vi "UHR-Fleezers Control (host) - 12.5.vi"() -> ()   [LabVIEW 2012] (continued)
        n1392 = Multiply(x=w2006, y=3.2767) -> (x*y=w2005:dbl)
        n1393 = local read "Green Intensity % (FB OFF)"() -> (w2009:dbl)
        n1394 = Multiply(x=w2009, y=655.35) -> (x*y=w2010:dbl)
        n1395 = To Unsigned Word Integer(number=w2010) -> (unsigned 16bit integer=w2008:u16)
        n1396 = local read "Green int current ON count adj"() -> (w2012:u32)
        n1397 = local read "Laser interlacing mode"() -> (w2002:enum32{"Laser ON", "Laser OFF", "Interlace"})
        n1398 = local read "Green FB Gains"() -> (w1999:T9)
        n1399 = local read "Green Laser ON"() -> (w2003:bool)
        n1400 = local read "Green FB On/Off"() -> (w2013:bool)
        n1401 = Equal?(x=w2002, y=enum32{"Laser ON", "Laser OFF", "Interlace"}."Interlace") -> (x = y?=w2000:bool)
        n1402 = Unbundle By Name(w1999) -> ("proportional gain (Kc)"=w1998:i16, "integral gain (Kc*Ts/Ti)"=w1997:i16, "derivative gain (Kc*Td/Ts)"=w1996:i16)
        n1403 = Compound Arithmetic op=AND(w2000, w2013, w2003) -> (w2004:bool)
        n1404 = xnode "Read/Write Control"("FPGA VI Reference In"=w2016, "error in"=w2015, "Green FB Setpoint"=w2005, "Green FB On/Off"=w2004, "Current Out"=w2008, "Green int current ON count adj"=w2012, "P3"=w1998, "I3"=w1997, "D3"=w1996) -> ("error out"=w2014:errorcluster)  [unwired: 1 out]
      }
      event "Blue FB Setpoint (mV)", "Blue FB Gains", "Blue FB On/Off", "Blue Intensity % (FB OFF)", "Blue int AO ON count adjust": Value Change {
        # "16 bit analog out"
        n1405 = event-data() -> ()  [unwired: 7 out]
        n1406 = Multiply(x="Blue FB Setpoint (mV)", y=3.2767) -> (x*y=w2030:dbl)
        n1407 = Multiply(x="Blue Intensity % (FB OFF)", y=655.35) -> (x*y=w2033:dbl)
        n1408 = To Unsigned Word Integer(number=w2033) -> (unsigned 16bit integer=w2032:u16)
        n1409 = local read "Laser interlacing mode"() -> (w2028:enum32{"Laser ON", "Laser OFF", "Interlace"})
        n1410 = Unbundle By Name("Blue FB Gains") -> ("proportional gain (Kc)"=w2025:i16, "integral gain (Kc*Ts/Ti)"=w2024:i16, "derivative gain (Kc*Td/Ts)"=w2023:i16)
        n1411 = local read "Blue Laser ON"() -> (w2017:bool)
        n1412 = Equal?(x=w2028, y=enum32{"Laser ON", "Laser OFF", "Interlace"}."Interlace") -> (x = y?=w2026:bool)
        n1413 = Compound Arithmetic op=AND(w2026, "Blue FB On/Off", w2017) -> (w2029:bool)
        n1414 = xnode "Read/Write Control"("FPGA VI Reference In"=w2037, "error in"=w2036, "Blue FB Setpoint"=w2030, "Blue FB On/Off"=w2029, "BI Current Out"=w2032, "Blue current ON count adj (AO)"="Blue int AO ON count adjust", "P5"=w2025, "I5"=w2024, "D5"=w2023) -> ("error out"=w2035:errorcluster)  [unwired: 1 out]
      }
      event "Red FB Setpoint (mV)", "Red FB Gains", "Red FB On/Off", "Red Intensity % (FB OFF)", "Red int current ON count adj": Value Change {
        n1415 = event-data() -> ()  [unwired: 7 out]
        n1416 = local read "Red FB Setpoint (mV)"() -> (w2049:dbl)
        n1417 = Multiply(x=w2049, y=3.2767) -> (x*y=w2048:dbl)
        n1418 = local read "Red Intensity % (FB OFF)"() -> (w2038:dbl)
        n1419 = Multiply(x=w2038, y=655.35) -> (x*y=w2052:dbl)
        n1420 = To Unsigned Word Integer(number=w2052) -> (unsigned 16bit integer=w2051:u16)
        n1421 = local read "Red int current ON count adj"() -> (w2054:u16)
        n1422 = local read "Laser interlacing mode"() -> (w2045:enum32{"Laser ON", "Laser OFF", "Interlace"})
        n1423 = local read "Red FB Gains"() -> (w2042:T9)
        n1424 = local read "Red Laser ON"() -> (w2046:bool)
        n1425 = local read "Red FB On/Off"() -> (w2055:bool)
        n1426 = Equal?(x=w2045, y=enum32{"Laser ON", "Laser OFF", "Interlace"}."Interlace") -> (x = y?=w2043:bool)
        n1427 = Unbundle By Name(w2042) -> ("proportional gain (Kc)"=w2041:i16, "integral gain (Kc*Ts/Ti)"=w2040:i16, "derivative gain (Kc*Td/Ts)"=w2039:i16)
        n1428 = Compound Arithmetic op=AND(w2043, w2055, w2046) -> (w2047:bool)
        n1429 = xnode "Read/Write Control"("FPGA VI Reference In"=w2058, "error in"=w2057, "Red FB Setpoint"=w2048, "Red FB On/Off"=w2047, "RI Current Out"=w2051, "Red int current ON count adj"=w2054, "P4"=w2041, "I4"=w2040, "D4"=w2039) -> ("error out"=w2056:errorcluster)  [unwired: 1 out]
      }
      event "+ phase (APD 1 Gate)", "- phase (APD 1 Gate)", "+ phase (APD 2 Gate)", "- phase (APD 2 Gate)", "+ phase (APD 3 Gate)", "- phase (APD 3 Gate)", "+ phase (APD Acq)", "- phase (APD Acq)": Value Change {
        n1430 = event-data() -> ()  [unwired: 7 out]
        n1431 = local read "Phase Adj. (APD 1 Gate)"() -> (w2078:i16)
        n1432 = Or(x="- phase (APD 1 Gate)", y="+ phase (APD 1 Gate)") -> (x .or. y?=w2080:bool)
        n1433 = Negate(x=w2078) -> (-x=w2085:i16)
        n1434 = Select(t=w2085, s="+ phase (APD 1 Gate)", f=w2078) -> (s? t:f=w2084:i16)
        n1435 = local read "Phase Adj. (APD 2 Gate)"() -> (w2075:i16)
        n1436 = Or(x="- phase (APD 2 Gate)", y="+ phase (APD 2 Gate)") -> (x .or. y?=w2073:bool)
        n1437 = Negate(x=w2075) -> (-x=w2077:i16)
        n1438 = Select(t=w2077, s="+ phase (APD 2 Gate)", f=w2075) -> (s? t:f=w2074:i16)
        n1439 = Negate(x="Phase Adj. (APD 3 Gate)") -> (-x=w2072:i16)
        n1440 = Or(x="- phase (APD 3 Gate)", y="+ phase (APD 3 Gate)") -> (x .or. y?=w2068:bool)
        n1441 = Select(t=w2072, s="+ phase (APD 3 Gate)", f="Phase Adj. (APD 3 Gate)") -> (s? t:f=w2069:i16)
        n1442 = local read "Phase Adj. (APD Acq)"() -> (w2066:i16)
        n1443 = Or(x="- phase (APD Acq)", y="+ phase (APD Acq)") -> (x .or. y?=w2064:bool)
        n1444 = Negate(x=w2066) -> (-x=w2067:i16)
        n1445 = Select(t=w2067, s="+ phase (APD Acq)", f=w2066) -> (s? t:f=w2065:i16)
        n1446 = xnode "Read/Write Control"("FPGA VI Reference In"=w2087, "error in"=w2086, "Phase count adjustment (APD 1 Gate)"=w2084, "Phase count adjustment (APD 2 Gate)"=w2074, "Phase count adjustment (APD 3 Gate)"=w2069, "Phase Count Adjustment (APD Acq)"=w2065) -> ("FPGA VI Reference Out"=w2082:T20, "error out"=w2083:errorcluster)
        n1447 = xnode "Read/Write Control"("FPGA VI Reference In"=w2082, "error in"=w2083, "+ phase (APD 1 Gate)"=w2080, "+ phase (APD 2 Gate)"=w2073, "+ phase (APD 3 Gate)"=w2068, "+ phase (APD Acq)"=w2064) -> ("error out"=w2081:errorcluster)  [unwired: 1 out]
      }
      event "Invert APD Gate", "APD Gate ON Count", "APD Gate OFF Count", "APD Gate", "APD Integration Time (s)", "APD AO Scale Factor", "Duty Frequency (ON 1/N cycles)", "Interlace ON count", "Interlace OFF count": Value Change {
        n1448 = event-data() -> ()  [unwired: 7 out]
        n1449 = Add(x="Interlace ON count", y="Interlace OFF count") -> (x+y=w2093:u16)
        n1450 = Add(x="APD Gate ON Count", y="APD Gate OFF Count") -> (x+y=w2104:u16)
        n1451 = Multiply(x="Duty Frequency (ON 1/N cycles)", y=w2093) -> (x*y=w2089:u16)
        "Green AI Count" <- w2089
        "Red AI Count" <- w2089
        "Blue AI Count" <- w2089
        n1452 = Subtract(x=w2089, y="Interlace ON count") -> (x-y=w2092:u16)
        n1453 = Multiply(x=w2104, y="Duty Frequency (ON 1/N cycles)") -> (x*y=w2103:u16)
        n1454 = Subtract(x=w2103, y="APD Gate ON Count") -> (x-y=w2102:u16)
        n1455 = local read "DMA Update Period (s)"() -> (w2105:dbl)
        n1456 = Multiply(x="APD Integration Time (s)", y=40000000.0) -> (x*y=w2109:dbl)
        n1457 = Reciprocal(x="APD Integration Time (s)") -> (1/x=→"APD Acq Rate (Hz)":dbl)
        n1458 = To Unsigned Long Integer(number=w2109) -> (unsigned 32bit integer=w2095:u32)
        "APD Int. Count" <- w2095
        n1459 = local read "Number of APDs"() -> (w2088:u8)
        n1460 = Divide(x=w2105, y="APD Integration Time (s)") -> (x/y=w2107:dbl)
        n1461 = Multiply(x=w2088, y=w2107) -> (x*y=w2106:dbl)
        n1462 = local write "APD Samples/FIFO Acq."(w2107) -> ()
        n1463 = local write "APD Elements/DMA read"(w2106) -> ()
        n1464 = xnode "Read/Write Control"("FPGA VI Reference In"=w2113, "error in"=w2112, "Invert APD Gate"="Invert APD Gate", "APD Gate ON Count"="APD Gate ON Count", "APD Gate OFF Count"=w2102, "APD Acq Rate Count"=w2095, "APD Gate Operating Mode"="APD Gate", "APD AO scale factor"="APD AO Scale Factor", "Green interlace ON count"="Interlace ON count", "Green interlace OFF count"=w2092, "Green interlace ON count 2"="Interlace ON count", "Green interlace OFF count 2"=w2092, "Green FB Count"=w2089, "Red interlace ON count"="Interlace ON count", "Red interlace OFF count"="Interlace OFF count", "Red FB Count"=w2089, "Red interlace ON count 2"="Interlace ON count", "Red interlace OFF count 2"="Interlace OFF count", "Blue ON count (AO)"="Interlace ON count", "Blue OFF count (AO)"="Interlace OFF count", "Blue interlace OFF count (D)"="Interlace OFF count", "Blue interlace ON count (D)"="Interlace ON count", "Blue Int Count"=w2089) -> ("error out"=w2111:errorcluster)  [unwired: 1 out]
      }
      event "Neg. TTrig FPGA": Value Change {
        n1465 = event-data() -> ()  [unwired: 7 out]
        n1466 = xnode "Read/Write Control"("FPGA VI Reference In"=w2116, "error in"=w2115, "TTrig Negate Pos"="Neg. TTrig FPGA") -> ()  [unwired: 2 out]
      }
      event "Test ttrig": Value Change {
        n1467 = event-data() -> ()  [unwired: 7 out]
        n1468 = xnode "Read/Write Control"("FPGA VI Reference In"=w2120, "error in"=w2119, "TTrig?"=TRUE) -> ("error out"=w2118:errorcluster)  [unwired: 1 out]
      }
      event "Number of F/B Scans (AOD)", "Scan Speed (nm/s)", "Scan BD", "Initial delta (MHz)", "Step Size (nm)", "Scan Range (nm)": Value Change {
        w2183 = 123.0  # AOM cal (nm/MHz)
        n1469 = event-data() -> ()  [unwired: 7 out]
        n1470 = local read "BD 1 Frequency 1 (MHz)"() -> (w2166:dbl)
        n1471 = local read "AOM X Cal (nm/MHz)"() -> (w2158:dbl)
        n1472 = local read "X RF Frequency Limits (MHz)"() -> (w2170:T16)
        n1473 = local read "Y RF Frequency Limits (MHz)"() -> (w2167:T16)
        n1474 = local read "BD 2 Frequency 1 (MHz)"() -> (w2172:dbl)
        n1475 = Negate(x="Scan Range (nm)") -> (-x=w2136:dbl)
        n1476 = Divide(x=w2136, y=w2158) -> (x/y=w2140:dbl)
        n1477 = Select(t=w2170, s="Scan BD", f=w2167) -> (s? t:f=w2169:T16)
        n1478 = Select(t=w2166, s="Scan BD", f=w2172) -> (s? t:f=w2171:dbl)
        n1479 = Unbundle By Name(w2169) -> ("Maximum"=w2178:dbl, "Minimum"=w2177:dbl)
        n1480 = Add(x=w2140, y=w2171) -> (x+y=w2175:dbl)
        n1481 = Divide(x=w2136, y="Step Size (nm)") -> (x/y=w2155:dbl)
        n1482 = Divide(x="Step Size (nm)", y=w2158) -> (x/y=w2164:dbl)
        n1483 = Absolute Value(x=w2155) -> (abs(x)=w2139:dbl)
        n1484 = Sign(1:w2136) -> (0:w2137:dbl)
        n1485 = In Range and Coerce(upper limit=w2178, x=w2175, lower limit=w2177) -> (coerced(x)=w2174:dbl, In Range?=w2176:bool)
        n1486 = To Unsigned Quad Integer(1:w2139) -> (0:w2154:u64)
        "Scan steps (AOD)" <- w2154
        n1487 = call "IR AOM freq to word.vi"("Frequency In (MHz)"=w2164) -> ("Frequency Word Out (double)"=w2161:dbl)
        n1488 = Multiply(x=w2137, y=w2161) -> (x*y=w2138:dbl)
        n1489 = Subtract(x=w2175, y=w2174) -> (x-y=w2173:dbl)
        n1490 = To Quad Integer(1:w2138) -> (0:w2160:i64)
        "Incr. int (AOD)" <- w2160
        n1491 = Subtract(x=w2140, y=w2173) -> (x-y=w2159:dbl)
        "Scan Range (MHz)" <- w2159
        n1492 = Select(t=w2140, s=w2176, f=w2159) -> (s? t:f=w2179:dbl)
        n1493 = Multiply(x=w2159, y=w2158) -> (x*y=w2157:dbl)
        n1494 = Decrement(x=w2154) -> (x-1=w2207:u64)
        n1495 = Negate(x=w2157) -> (-x=w2153:dbl)
        n1496 = local write "Scan Range (nm)"(w2153) -> ()
        n1497 = Divide(x=w2179, y=w2207) -> (x/y=w2163:dbl)
        "Scan Increment (MHz)" <- w2163
        n1498 = call "IR AOM freq to word.vi"("Frequency In (MHz)"=w2163) -> ("Frequency Word Out (double)"=w2162:dbl)
        n1499 = Divide(x="Step Size (nm)", y="Scan Speed (nm/s)") -> (x/y=w2150:dbl)
        n1500 = To Quad Integer(1:w2162) -> ()  [unwired: 1 out]
        n1501 = local read "Number Interlace Sets"() -> (w2134:u8)
        n1502 = local read "AI Count (ticks)"() -> (w2135:u16)
        n1503 = local read "Total Counts (ticks)"() -> (w2133:u16)
        n1504 = local read "# Samples/trap"() -> (w2165:u32)
        n1505 = Multiply(x=w2135, y=w2134) -> (x*y=w2132:u16)
        n1506 = Divide(x=w2133, y=w2132) -> (x/y=w2131:dbl)
        n1507 = Select(t=w2166, s="Scan BD", f=w2172) -> (s? t:f=w2204:dbl)
        "Initial freq. (MHz)" <- w2204
        n1508 = Add(x=w2179, y=w2204) -> (x+y=→"Final freq. (MHz)":dbl)
        n1509 = Divide(x=w2133, y=40000000.0) -> (x/y=w2149:dbl)
        n1510 = Divide(x=w2150, y=w2149) -> (x/y=w2148:dbl)
        n1511 = To Unsigned Quad Integer(1:w2148) -> (0:w2123:u64)
        n1512 = Quotient & Remainder(x=w2123, y=u64 2) -> (x-y*floor(x/y)=w2127:u64)  [unwired: 1 out]
        n1513 = Equal?(x=w2127, y=u64 0) -> (x = y?=w2125:bool)
        n1514 = Decrement(x=w2123) -> (x-1=w2124:u64)
        n1515 = Select(t=w2123, s=w2125, f=w2124) -> (s? t:f=w2122:u64)
        "Cycles/step (AOD)" <- w2122
        n1516 = xnode "Read/Write Control"("FPGA VI Reference In"=w2215, "error in"=w2214, "Scan steps"=w2154, "Number of scans"="Number of F/B Scans (AOD)", "Cycles per step"=w2122, "Scan freq.  increment"=w2160, "Scan BD"="Scan BD") -> ("error out"=w2213:errorcluster)  [unwired: 1 out]
        n1517 = Multiply(x=w2154, y=w2122) -> (x*y=w2208:u64)
        n1518 = Multiply(x=w2208, y=u64 2) -> (x*y=w2130:u64)
        n1519 = Multiply(x=w2131, y=w2130) -> (x*y=w2129:dbl)
        "Data points/scan (f/b)" <- w2129
        n1520 = Multiply(x=w2129, y="Number of F/B Scans (AOD)") -> (x*y=w2211:dbl)
        "Data points/scans" <- w2211
        n1521 = Divide(x=w2211, y=w2165) -> (x/y=→"N sets should be saved":dbl)
        n1522 = Multiply(x=w2208, y=w2149) -> (x*y=w2147:dbl)
        "Time/Scan (s) (AOD)" <- w2147
        n1523 = Select(t=w2179, s="Scan BD", f=0.0) -> (s? t:f=w2205:dbl)
        n1524 = Select(t=0.0, s="Scan BD", f=w2179) -> (s? t:f=w2201:dbl)
        n1525 = local read "BD 2 Frequency 2 (MHz)"() -> (w2197:dbl)
        n1526 = local read "BD 1 Frequency 2 (MHz)"() -> (w2200:dbl)
        n1527 = Add(x=w2201, y=w2172) -> (x+y=w2198:dbl)
        n1528 = Add(x=w2166, y=w2205) -> (x+y=w2199:dbl)
        n1529 = Multiply(x=w2147, y=2.0) -> (x*y=w2146:dbl)
        n1530 = Multiply(x=w2146, y="Number of F/B Scans (AOD)") -> (x*y=w2143:dbl)
        n1531 = Divide(x=w2143, y=60.0) -> (x/y=→"Time to Finish All (min)":dbl)
        n1532 = Add(x="Trap 2 Bead Size (nm)", y="Trap 1 Bead Size (nm)") -> (x+y=w2187:dbl)
        n1533 = Divide(x=w2187, y=2.0) -> (x/y=w2181:dbl)
        n1534 = local read "Initial delta (MHz)"() -> (w2184:dbl)
        n1535 = Subtract(x=w2198, y=w2197) -> (x-y=w2195:dbl)
        n1536 = Subtract(x=w2199, y=w2200) -> (x-y=w2196:dbl)
        n1537 = Square(x=w2195) -> (x^2=w2194:dbl)
        n1538 = Square(x=w2196) -> (x^2=w2193:dbl)
        n1539 = Add(x=w2193, y=w2194) -> (x+y=w2192:dbl)
        n1540 = Square Root(x=w2192) -> (sqrt(x)=w2191:dbl)
        "Final delta (MHz)" <- w2191
        n1541 = Multiply(x=w2183, y=w2191) -> (x*y=w2190:dbl)
        n1542 = Multiply(x=w2184, y=w2183) -> (x*y=w2182:dbl)
        n1543 = Subtract(x=w2182, y=w2181) -> (x-y=→"Initial sep (nm)":dbl)
        n1544 = Subtract(x=w2190, y=w2181) -> (x-y=→"Final sep (nm)":dbl)
      }
      event "Freq or Amp switch first", "Swap F1 and F2", "Freq switch delay", "Amp switch delay": Value Change {
        n1545 = event-data() -> ()  [unwired: 7 out]
        n1546 = local read "Amp switch delay"() -> (w2216:u16)
        n1547 = local read "Swap F1 and F2"() -> (w2217:bool)
        n1548 = xnode "Read/Write Control"("FPGA VI Reference In"=w2220, "error in"=w2219, "Swap F1 and F2"=w2217, "Amp switch delay"=w2216) -> ("error out"=w2218:errorcluster)  [unwired: 1 out]
      }
      event "Scan steps (MCL)", "Number of scans (MCL)", "Scan Range (V)\n(of steps)", "2D or 1D Scan", "N APD Samp/step", "Fast Scan Dir", "Continuous MCL Scanning", "Scan lines (y)": Value Change {
        w2222 = 32767.0 ("y")
        n1549 = event-data() -> ()  [unwired: 7 out]
        n1550 = Select(t="Scan lines (y)", s="2D or 1D Scan", f="Number of scans (MCL)") -> (s? t:f=w2227:u64)
        n1551 = Decrement(x="Scan steps (MCL)") -> (x-1=w2243:u64)
        n1552 = Divide(x="Scan Range (V)\n(of steps)", y=w2243) -> (x/y=w2242:dbl)
        "Desired Scan Incr (V)" <- w2242
        n1553 = local read "APD Integration Time (s)"() -> (w2235:dbl)
        n1554 = Multiply(x=w2242, y=w2222) -> (x*y=w2251:dbl)
        n1555 = Divide(x=w2251, y=10.0) -> (x/y=w2241:dbl)
        "Desired incr (int)" <- w2241
        n1556 = local read "Update Count (MCL)"() -> (w2247:u32)
        n1557 = Round Toward -Infinity(1:w2241) -> (0:w2250:dbl)
        n1558 = To Word Integer(number=w2250) -> (16bit integer=w2225:i16)
        "Actual Incr. int (MCL)" <- w2225
        n1559 = Multiply(x=w2235, y=40000000.0) -> (x*y=w2248:dbl)
        n1560 = Divide(x=w2248, y=w2247) -> (x/y=w2246:dbl)
        n1561 = Multiply(x=i16 10, y=w2225) -> (x*y=w2223:i16)
        n1562 = Multiply(x="N APD Samp/step", y=w2246) -> (x*y=w2245:dbl)
        "Cycles/step (MCL)" <- w2245
        n1563 = Divide(x=w2223, y=w2222) -> (x/y=→"Actual MCL Inc (V)":dbl)
        n1564 = Multiply(x="N APD Samp/step", y="Scan steps (MCL)") -> (x*y=w2237:dbl)
        n1565 = local read "APD Samples/FIFO Acq."() -> (w2234:dbl)
        n1566 = Multiply(x=w2237, y=u64 2) -> (x*y=w2236:dbl)
        "Data points/scan (f+b)" <- w2236
        n1567 = Multiply(x=w2236, y=w2227) -> (x*y=w2254:dbl)
        "Data points/scans (MCL)" <- w2254
        n1568 = Multiply(x=w2235, y=w2236) -> (x*y=w2228:dbl)
        "Time/f+b scan (s) (MCL)" <- w2228
        n1569 = Divide(x=w2254, y=w2234) -> (x/y=→"N sets should be saved (MCL)":dbl)
        n1570 = Multiply(x=w2228, y=w2227) -> (x*y=→"Total Time (s)":dbl)
        n1571 = Not(x="Fast Scan Dir") -> (.not. x?=w2232:bool)
        n1572 = xnode "Read/Write Control"("FPGA VI Reference In"=w2258, "error in"=w2257, "Scan steps (MCL)"="Scan steps (MCL)", "Number of scans (MCL)"=w2227, "Cycles per step (MCL)"=w2245, "Scan freq.  increment (MCL)"=w2225, "1D or 2D Scan?"="2D or 1D Scan", "MCL Scan Axis"=w2232, "Cont. Scan (MCL)"="Continuous MCL Scanning") -> ("error out"=w2256:errorcluster)  [unwired: 1 out]
      }
      event "Read Cal": Value Change {
        w2260 = 1000.0 ("y")
        n1573 = event-data() -> ()  [unwired: 7 out]
        n1574 = local read "Save file name"() -> (w2285:path)
        n1575 = local write "Read Cal"(FALSE ("Read Cal")) -> ()
        n1576 = Strip Path(path=w2285) -> (stripped path=w2284:path)  [unwired: 1 out]
        n1577 = Path To String(path=w2284) -> (string=w2283:string)
        n1578 = Concatenate Strings(w2283, "\\current.cal" ("string")) -> (w2281:string)
        n1579 = String To Path(string=w2281) -> (path=w2280:path)
        n1580 = Open/Create/Replace File(file path (use dialog)=w2280, operation (0:open)=T28."open", access (0:read/write)=enum16{"read/write", "read-only", "write-only"}."read-only") -> (refnum out=w2288:refnum<file>, error out=w2274:errorcluster)  [unwired: 1 in, 3 out]
        n1581 = Deny Access(4:w2274, 7:w2288) -> (0:w2273:errorcluster, 3:w2279:refnum<file>)  [unwired: 1 out]
        n1582 = Read from Binary File(5:0.0, 8:w2273, 9:T27."big-endian, network order" ("byte order (0:big-endian, network order)"), 10:-1 ("count (1)"), 11:w2279) -> (0:w2272:errorcluster, 2:w2270:dbl[], 3:w2275:refnum<file>)  [unwired: 2 out]
        n1583 = Array To Cluster(array=w2270) -> (cluster=w2269:T30)
        n1584 = Unbundle(w2269) -> ("[0]"=w2268:dbl, "[1]"=w2267:dbl, "[2]"=w2266:dbl, "[3]"=w2265:dbl, "[4]"=w2264:dbl, "[5]"=w2263:dbl)
        n1585 = Close File(refnum=w2275, error in=w2272) -> (error out=→"Read cal error":errorcluster)  [unwired: 1 out]
        n1586 = Multiply(x=w2263, y=w2260) -> (x*y=w2261:dbl)
        n1587 = local write "T2 kappa_x (pN/nm)"(w2265) -> ()
        n1588 = local write "T1 kappa_x (pN/nm)"(w2266) -> ()
        n1589 = local write "T1 alpha_x (nm/V)"(w2268) -> ()
        n1590 = local write "T2 alpha_x (nm/V)"(w2267) -> ()
        n1591 = Multiply(x=w2264, y=w2260) -> (x*y=w2262:dbl)
        n1592 = local write "T1 offset_x (mV)"(w2262) -> ()
        n1593 = local write "T2 offset_x (mV)"(w2261) -> ()
      }
      event "Abort MCL Scan": Value Change {
        n1594 = event-data() -> ()  [unwired: 7 out]
        n1595 = local write "MCL Scanning"(FALSE ("MCL Scanning")) -> ()
        n1596 = xnode "Read/Write Control"("FPGA VI Reference In"=w2293, "error in"=w2292, "Abort scan (MCL)"="Abort MCL Scan") -> ("error out"=w2291:errorcluster)  [unwired: 1 out]
      }
      event "Update Count (MCL)": Value Change {
        n1597 = event-data() -> ()  [unwired: 7 out]
        n1598 = xnode "Read/Write Control"("FPGA VI Reference In"=w2297, "error in"=w2296, "MCL count"="Update Count (MCL)") -> ("error out"=w2295:errorcluster)  [unwired: 1 out]
      }
      event "+ phase (MCL)", "- phase (MCL)": Value Change {
        n1599 = event-data() -> ()  [unwired: 7 out]
        n1600 = Or(x="- phase (MCL)", y="+ phase (MCL)") -> (x .or. y?=w2300:bool)
        n1601 = Negate(x="Phase adjust (MCL)") -> (-x=w2306:i16)
        n1602 = Select(t=w2306, s="+ phase (MCL)", f="Phase adjust (MCL)") -> (s? t:f=w2304:i16)
        n1603 = xnode "Read/Write Control"("FPGA VI Reference In"=w2308, "error in"=w2307, "Phase count adjustment (MCL)"=w2304) -> ("FPGA VI Reference Out"=w2301:T20, "error out"=w2302:errorcluster)
        n1604 = xnode "Read/Write Control"("FPGA VI Reference In"=w2301, "error in"=w2302, "+ phase (MCL)"=w2300) -> ("error out"=w2299:errorcluster)  [unwired: 1 out]
      }
      event "Abort AOD Scan": Value Change {
        n1605 = event-data() -> ()  [unwired: 7 out]
        n1606 = xnode "Read/Write Control"("FPGA VI Reference In"=w2312, "error in"=w2311, "Abort scan"="Abort AOD Scan") -> ("error out"=w2310:errorcluster)  [unwired: 1 out]
      }
      event "Continuous AOD Scanning": Value Change {
        n1607 = event-data() -> ()  [unwired: 7 out]
        n1608 = xnode "Read/Write Control"("FPGA VI Reference In"=w2316, "error in"=w2315, "Cont. Scan"="Continuous AOD Scanning") -> ("error out"=w2314:errorcluster)  [unwired: 1 out]
      }
      event "Index": Value Change {
        n1609 = event-data() -> ()  [unwired: 7 out]
        n1610 = call "Create new save file.vi"("Insert"="", "Ext"=".dat" ("string"), "Index In"="Index") -> ("Path Out"=→"Save file name":path, "Index Out"=w2317:dbl)
        "Save index" <- w2317
        n1611 = local write "Index"(w2317) -> ()
      }
      event "AO1", "AO2": Value Change {
        w2332 = 10.0 ("y")
        w2331 = 32767.0 ("y")
        n1612 = event-data() -> ()  [unwired: 7 out]
        n1613 = local read "AO2"() -> (w2330:dbl)
        n1614 = local read "AO1"() -> (w2327:dbl)
        n1615 = Multiply(x=w2327, y=w2331) -> (x*y=w2326:dbl)
        n1616 = Multiply(x=w2330, y=w2331) -> (x*y=w2329:dbl)
        n1617 = Divide(x=w2326, y=w2332) -> (x/y=w2325:dbl)
        n1618 = Divide(x=w2329, y=w2332) -> (x/y=w2328:dbl)
        n1619 = To Word Integer(number=w2325) -> (16bit integer=w2333:i16)
        n1620 = To Word Integer(number=w2328) -> (16bit integer=w2334:i16)
        n1621 = xnode "Read/Write Control"("FPGA VI Reference In"=w2324, "error in"=w2323, "AO1"=w2333, "AO2"=w2334) -> ("error out"=w2322:errorcluster)  [unwired: 1 out]
      }
      event "Inject Pump 1": Value Change {
        n1622 = event-data() -> ()  [unwired: 7 out]
        n1623 = local read "Use Harvard pumps\nfor beads (else Chemyx)"() -> (w2336:bool)
        n1624 = case shown="True" w2336 {
          tunnel: "Inject Pump 1" -> [w2340 w2378]
          tunnel: w2335 -> [_ w2379]
          frame False {
            n1625 = local read "Pump write delay (ms)"() -> (w2339:dbl)
            n1626 = local read "Chemyx Syringe Pump Serial Port"() -> (w2338:refnum<visa-resource-name>)
            n1627 = case shown="True" w2340 {
              tunnel: w2339 -> [w2346 w2360]
              tunnel: w2338 -> [w2343 w2359]
              frame False {
                n1628 = flat-sequence {
                  tunnel: w2343 -> [w2347]
                  tunnel: [w2347] -> w2344
                  tunnel: w2346 -> [_]
                  tunnel: [w2350] -> w2345
                  tunnel: w2344 -> [w2350]
                  tunnel: w2345 -> [w2351]
                  tunnel: [w2351] -> w2341
                  tunnel: [w2353] -> w2342
                  tunnel: w2341 -> [w2353]
                  tunnel: w2342 -> [w2355]
                  frame #0 {
                    n1629 = call "Write to pump.vi"("string"="enter pump1", "VISA resource name"=w2347) -> ()  [unwired: 1 out]
                  }
                  frame #1 {
                    n1630 = Wait (ms)(milliseconds to wait="Pump pause delay (ms)") -> ()  [unwired: 1 out]
                  }
                  frame #2 {
                    n1631 = call "Write to pump.vi"("string"="stop", "VISA resource name"=w2351) -> ()  [unwired: 1 out]
                  }
                  frame #3 {
                    n1632 = Wait (ms)(milliseconds to wait=u32 500) -> ()  [unwired: 1 out]
                  }
                  frame #4 {
                    n1633 = call "Write to pump.vi"("string"="stop", "VISA resource name"=w2355) -> ()  [unwired: 1 out]
                  }
                }
              }
              frame True {
                n1634 = flat-sequence {
                  tunnel: w2359 -> [w2369]
                  tunnel: w2360 -> [w2364]
                  tunnel: w2360 -> [w2371]
                  tunnel: w2359 -> [w2372]
                  tunnel: [w2372] -> w2357
                  tunnel: [w2374] -> w2358
                  tunnel: w2357 -> [w2374]
                  tunnel: w2358 -> [w2376]
                  frame #0 {
                    n1635 = local read "All Pump Parameters"() -> (w2363:T5)
                    n1636 = Unbundle By Name(w2363) -> ("Pump 1"=w2370:T31)
                    n1637 = call "Set pump parameters.vi"("Pump write delay (ms)"=w2364, "Volume (uL)"="Ch 1 Inject Volume (uL)", "Rate (uL/h)"="Ch 1 Inject Rate (ul/h)", "Units"=4.0, "Pump #"=1.0, "Pump Parameters In"=w2370, "VISA resource name"=w2369) -> ("Pump Parameters Out"=w2362:T31)  [unwired: 3 in]
                    n1638 = Bundle By Name(cluster=w2363, "Pump 1"=w2362) -> (w2361:T5)
                    n1639 = local write "All Pump Parameters"(w2361) -> ()
                  }
                  frame #1 {
                    n1640 = Wait (ms)(milliseconds to wait=w2371) -> ()  [unwired: 1 out]
                  }
                  frame #2 {
                    n1641 = call "Write to pump.vi"("string"="start", "VISA resource name"=w2372) -> ()  [unwired: 1 out]
                  }
                  frame #3 {
                    n1642 = Wait (ms)(milliseconds to wait=u32 500) -> ()  [unwired: 1 out]
                  }
                  frame #4 {
                    n1643 = call "Write to pump.vi"("string"="start", "VISA resource name"=w2376) -> ()  [unwired: 1 out]
                  }
                }
              }
            }
          }
          frame True {
            n1644 = case shown="False" w2378 {
              tunnel: w2379 -> [w2380 w2390]
              frame False {
                n1645 = flat-sequence {
                  tunnel: w2380 -> [w2382]
                  frame #0 {
                    n1646 = local write "Flushing P1"(FALSE ("Flushing P1")) -> ()
                    n1647 = Concatenate Strings("stop" ("string"), "\r") -> (w2384:string)
                    n1648 = VISA Write(VISA resource name=w2382, write buffer=w2384) -> ()  [unwired: 1 in, 3 out]
                  }
                  frame #1 {
                    n1649 = property on="Clear Volume P1" class="Bool (strict)"("Val(Sgnl)"=TRUE ("Value (Signaling)")) -> ()  [unwired: 2 in, 2 out]
                  }
                }
              }
              frame True {
                n1650 = local read "Normal Flow Rate (ul/h) P1"() -> (w2388:dbl)
                n1651 = Number To Decimal String(number=w2388) -> (decimal integer string=w2394:string)  [unwired: 1 in]
                n1652 = Concatenate Strings("irate  " ("string"), w2394, " u/h" ("string"), "\r") -> (w2392:string)
                n1653 = VISA Write(VISA resource name=w2390, write buffer=w2392) -> (VISA resource name out=w2389:refnum<visa-resource-name>)  [unwired: 1 in, 2 out]
                n1654 = Concatenate Strings("irun" ("string"), "\r") -> (w2396:string)
                n1655 = VISA Write(VISA resource name=w2389, write buffer=w2396) -> ()  [unwired: 1 in, 3 out]
              }
            }
          }
        }
      }
      event "Inject Pump 3": Value Change {
        n1656 = event-data() -> ()  [unwired: 7 out]
        n1657 = local read "Use Harvard pumps\nfor beads (else Chemyx)"() -> (w2399:bool)
        n1658 = case shown="True" w2399 {
          tunnel: "Inject Pump 3" -> [w2403 w2442]
          tunnel: w2398 -> [_ w2441]
          frame False {
            n1659 = local read "Pump write delay (ms)"() -> (w2402:dbl)
            n1660 = case shown="True" w2403 {
              tunnel: w2402 -> [w2409 w2423]
              tunnel: "Chemyx Syringe Pump Serial Port" -> [w2406 w2422]
              frame False {
                n1661 = flat-sequence {
                  tunnel: w2406 -> [w2410]
                  tunnel: [w2410] -> w2407
                  tunnel: w2409 -> [_]
                  tunnel: [w2413] -> w2408
                  tunnel: w2407 -> [w2413]
                  tunnel: w2408 -> [w2414]
                  tunnel: [w2414] -> w2404
                  tunnel: [w2416] -> w2405
                  tunnel: w2404 -> [w2416]
                  tunnel: w2405 -> [w2418]
                  frame #0 {
                    n1662 = call "Write to pump.vi"("string"="enter pump3", "VISA resource name"=w2410) -> ()  [unwired: 1 out]
                  }
                  frame #1 {
                    n1663 = local read "Pump pause delay (ms)"() -> (w2412:u32)
                    n1664 = Wait (ms)(milliseconds to wait=w2412) -> ()  [unwired: 1 out]
                  }
                  frame #2 {
                    n1665 = call "Write to pump.vi"("string"="stop", "VISA resource name"=w2414) -> ()  [unwired: 1 out]
                  }
                  frame #3 {
                    n1666 = Wait (ms)(milliseconds to wait=u32 0) -> ()  [unwired: 1 out]
                  }
                  frame #4 {
                    n1667 = call "Write to pump.vi"("string"="stop", "VISA resource name"=w2418) -> ()  [unwired: 1 out]
                  }
                }
              }
              frame True {
                n1668 = flat-sequence {
                  tunnel: w2422 -> [w2432]
                  tunnel: w2423 -> [w2427]
                  tunnel: w2423 -> [w2434]
                  tunnel: w2422 -> [w2435]
                  tunnel: [w2435] -> w2421
                  tunnel: [w2438] -> w2420
                  tunnel: w2421 -> [w2438]
                  tunnel: w2420 -> [w2439]
                  frame #0 {
                    n1669 = local read "All Pump Parameters"() -> (w2426:T5)
                    n1670 = Unbundle By Name(w2426) -> ("Pump 3"=w2433:T31)
                    n1671 = call "Set pump parameters.vi"("Pump write delay (ms)"=w2427, "Volume (uL)"="Ch 3 Inject Volume (uL)", "Rate (uL/h)"="Ch 3 Inject Rate (ul/h)", "Units"=4.0, "Pump #"=3.0, "Pump Parameters In"=w2433, "VISA resource name"=w2432) -> ("Pump Parameters Out"=w2425:T31)  [unwired: 3 in]
                    n1672 = Bundle By Name(cluster=w2426, "Pump 3"=w2425) -> (w2424:T5)
                    n1673 = local write "All Pump Parameters"(w2424) -> ()
                  }
                  frame #1 {
                    n1674 = Wait (ms)(milliseconds to wait=w2434) -> ()  [unwired: 1 out]
                  }
                  frame #2 {
                    n1675 = call "Write to pump.vi"("string"="start", "VISA resource name"=w2435) -> ()  [unwired: 1 out]
                  }
                  frame #3 {
                    n1676 = Wait (ms)(milliseconds to wait=u32 500) -> ()  [unwired: 1 out]
                  }
                  frame #4 {
                    n1677 = call "Write to pump.vi"("string"="start", "VISA resource name"=w2439) -> ()  [unwired: 1 out]
                  }
                }
              }
            }
          }
          frame True {
            n1678 = case shown="False" w2442 {
              tunnel: w2441 -> [w2443 w2450]
              frame False {
                n1679 = flat-sequence {
                  tunnel: w2443 -> [w2445]
                  frame #0 {
                    n1680 = local write "Flushing P3"(FALSE ("Flushing P3")) -> ()
                    n1681 = Concatenate Strings("stop" ("string"), "\r") -> (w2447:string)
                    n1682 = VISA Write(VISA resource name=w2445, write buffer=w2447) -> ()  [unwired: 1 in, 3 out]
                  }
                  frame #1 {
                    n1683 = property on="Clear Volume P3" class="Bool (strict)"("Val(Sgnl)"=TRUE ("Value (Signaling)")) -> ()  [unwired: 2 in, 2 out]
                  }
                }
              }
              frame True {
                n1684 = local read "Normal Flow Rate (ul/h) P3"() -> (w2451:dbl)
                n1685 = Number To Decimal String(number=w2451) -> (decimal integer string=w2457:string)  [unwired: 1 in]
                n1686 = Concatenate Strings("irate  " ("string"), w2457, " u/h" ("string"), "\r") -> (w2455:string)
                n1687 = VISA Write(VISA resource name=w2450, write buffer=w2455) -> (VISA resource name out=w2453:refnum<visa-resource-name>)  [unwired: 1 in, 2 out]
                n1688 = Concatenate Strings("irun" ("string"), "\r") -> (w2459:string)
                n1689 = VISA Write(VISA resource name=w2453, write buffer=w2459) -> ()  [unwired: 1 in, 3 out]
              }
            }
          }
        }
      }
      event "Inject Pump 2": Value Change {
        n1690 = event-data() -> ()  [unwired: 7 out]
        n1691 = local read "Pump write delay (ms)"() -> (w2463:dbl)
        n1692 = flat-sequence {
          tunnel: w2461 -> [w2476]
          tunnel: w2463 -> [w2472]
          tunnel: "Inject Pump 2" -> [_]
          tunnel: w2463 -> [w2478]
          tunnel: w2461 -> [w2479]
          frame #0 {
            n1693 = local read "All Pump Parameters"() -> (w2471:T5)
            n1694 = Multiply(x=60.0, y="Flush Center Ch Rate (ul/m)") -> (x*y=w2468:dbl)
            n1695 = Unbundle By Name(w2471) -> ("Pump 2"=w2477:T31)
            n1696 = call "Set pump parameters.vi"("Pump write delay (ms)"=w2472, "Volume (uL)"="Flush Center Ch Volume (uL)", "Rate (uL/h)"=w2468, "Units"=3.0, "Pump #"=2.0, "Pump Parameters In"=w2477, "VISA resource name"=w2476) -> ("Pump Parameters Out"=w2470:T31)  [unwired: 3 in]
            n1697 = Bundle By Name(cluster=w2471, "Pump 2"=w2470) -> (w2469:T5)
            n1698 = local write "All Pump Parameters"(w2469) -> ()
            n1699 = Add(x="Flush Center Ch Volume (uL)", y="Total Volume\nFlushed (uL)") -> (x+y=w2465:dbl)
            n1700 = local write "Total Volume\nFlushed (uL)"(w2465) -> ()
          }
          frame #1 {
            n1701 = Wait (ms)(milliseconds to wait=w2478) -> ()  [unwired: 1 out]
          }
          frame #2 {
            n1702 = call "Write to pump.vi"("string"="start", "VISA resource name"=w2479) -> ()  [unwired: 1 out]
          }
        }
        n1703 = local read "Chemyx Syringe Pump Serial Port"() -> (w2461:refnum<visa-resource-name>)
      }
      event "Sample Channel\nFlow": Value Change {
        n1704 = event-data() -> ()  [unwired: 7 out]
        n1705 = Select(t="irun" ("string"), s="Sample Channel\nFlow", f="stop" ("string")) -> (s? t:f=w2483:string)
        n1706 = Concatenate Strings(w2483, "\r") -> (w2486:string)
        n1707 = VISA Write(VISA resource name=w2481, write buffer=w2486) -> ()  [unwired: 1 in, 3 out]
      }
      event "Start Flow": Value Change {
        n1708 = event-data() -> ()  [unwired: 7 out]
        n1709 = local write "Sample Channel\nFlow"(TRUE ("Sample Channel\nFlow")) -> ()
        n1710 = local write "Start Flow"(FALSE ("Start Flow")) -> ()
        n1711 = Concatenate Strings("irun" ("string"), "\r") -> (w2492:string)
        n1712 = VISA Write(VISA resource name=w2488, write buffer=w2492) -> ()  [unwired: 1 in, 3 out]
      }
      event "Stop Flow": Value Change {
        w2494 = FALSE ("Stop Flow")
        n1713 = event-data() -> ()  [unwired: 7 out]
        n1714 = local write "Stop Flow"(w2494) -> ()
        n1715 = local write "Sample Channel\nFlow"(w2494) -> ()
        n1716 = Concatenate Strings("stop" ("string"), "\r") -> (w2497:string)
        n1717 = VISA Write(VISA resource name=w2495, write buffer=w2497) -> ()  [unwired: 1 in, 3 out]
      }
      event "Flow rate (uL/h)": Value Change {
        n1718 = event-data() -> ()  [unwired: 7 out]
        n1719 = Number To Decimal String(number="Flow rate (uL/h)") -> (decimal integer string=w2504:string)  [unwired: 1 in]
        n1720 = Concatenate Strings("irate  " ("string"), w2504, " u/h" ("string"), "\r") -> (w2503:string)
        n1721 = VISA Write(VISA resource name=w2500, write buffer=w2503) -> ()  [unwired: 1 in, 3 out]
      }
      event "Flush Sample": Value Change {
        n1722 = event-data() -> ()  [unwired: 7 out]
        n1723 = flat-sequence {
          tunnel: w2509 -> [w2537]
          tunnel: [w2517] -> w2508
          tunnel: [w2511] -> w2506
          tunnel: w2508 -> [w2541]
          tunnel: [w2541] -> w2507
          tunnel: w2506 -> [w2540]
          tunnel: w2507 -> [w2546]
          frame #0 {
            # "set paramaters (rate, volume) for flush, clear volume"
            n1724 = Number To Decimal String(number="Flush rate (uL/m)") -> (decimal integer string=w2533:string)  [unwired: 1 in]
            n1725 = Concatenate Strings("irate  " ("string"), w2533, " u/m" ("string"), "\r") -> (w2535:string)
            n1726 = VISA Write(VISA resource name=w2537, write buffer=w2535) -> (VISA resource name out=w2531:refnum<visa-resource-name>)  [unwired: 1 in, 2 out]
            n1727 = Reciprocal(x="Flush rate (uL/m)") -> (1/x=w2514:dbl)
            n1728 = Number To Decimal String(number="Volume (uL)") -> (decimal integer string=w2522:string)  [unwired: 1 in]
            n1729 = Multiply(x="Volume (uL)", y=w2514) -> (x*y=w2513:dbl)
            n1730 = Concatenate Strings("tvolume  " ("string"), w2522, " u" ("string"), "\r") -> (w2520:string)
            n1731 = Multiply(x=w2513, y=60000.0) -> (x*y=w2511:dbl)
            n1732 = VISA Write(VISA resource name=w2531, write buffer=w2520) -> (VISA resource name out=w2519:refnum<visa-resource-name>)  [unwired: 1 in, 2 out]
            n1733 = Concatenate Strings("cvolume" ("string"), "\r") -> (w2518:string)
            n1734 = VISA Write(VISA resource name=w2519, write buffer=w2518) -> (VISA resource name out=w2529:refnum<visa-resource-name>)  [unwired: 1 in, 2 out]
            n1735 = Concatenate Strings("irun" ("string"), "\r") -> (w2527:string)
            n1736 = VISA Write(VISA resource name=w2529, write buffer=w2527) -> (VISA resource name out=w2517:refnum<visa-resource-name>)  [unwired: 1 in, 2 out]
          }
          frame #1 {
            # "Have to wait until\nflow is done to reset\nrate"
            n1737 = Add(x=w2540, y=100.0) -> (x+y=w2539:dbl)
            n1738 = Wait (ms)(milliseconds to wait=w2539) -> ()  [unwired: 1 out]
          }
          frame #2 {
            # "reset flow rate to usual flow rate"
            n1739 = local read "Flow rate (uL/h)"() -> (w2552:dbl)
            n1740 = Number To Decimal String(number=w2552) -> (decimal integer string=w2550:string)  [unwired: 1 in]
            n1741 = Concatenate Strings("irate  " ("string"), w2550, " u/h" ("string"), "\r") -> (w2548:string)
            n1742 = VISA Write(VISA resource name=w2546, write buffer=w2548) -> (VISA resource name out=w2542:refnum<visa-resource-name>)  [unwired: 1 in, 2 out]
            n1743 = Concatenate Strings("cvolume" ("string"), "\r") -> (w2543:string)
            n1744 = VISA Write(VISA resource name=w2542, write buffer=w2543) -> ()  [unwired: 1 in, 3 out]
          }
        }
      }
      event "Flush Pump 3": Value Change {
        n1745 = event-data() -> ()  [unwired: 7 out]
        n1746 = flat-sequence {
          tunnel: w2553 -> [w2556]
          frame #0 {
            # "set paramaters (rate, volume) for flush, clear volume"
            n1747 = Number To Decimal String(number="Flush rate (uL/m) P3") -> (decimal integer string=w2578:string)  [unwired: 1 in]
            n1748 = local write "Inject Pump 3"(TRUE ("Inject Pump 3")) -> ()
            n1749 = Concatenate Strings("irate  " ("string"), w2578, " u/m" ("string"), "\r") -> (w2580:string)
            n1750 = VISA Write(VISA resource name=w2556, write buffer=w2580) -> (VISA resource name out=w2576:refnum<visa-resource-name>)  [unwired: 1 in, 2 out]
            n1751 = Reciprocal(x="Flush rate (uL/m) P3") -> (1/x=w2560:dbl)
            n1752 = Number To Decimal String(number="Volume (uL) P3") -> (decimal integer string=w2567:string)  [unwired: 1 in]
            n1753 = Multiply(x="Volume (uL) P3", y=w2560) -> (x*y=w2559:dbl)
            n1754 = Concatenate Strings("tvolume  " ("string"), w2567, " u" ("string"), "\r") -> (w2565:string)
            n1755 = Multiply(x=w2559, y=60.0) -> (x*y=→"HP3 Flush Time (s)":dbl)
            n1756 = VISA Write(VISA resource name=w2576, write buffer=w2565) -> (VISA resource name out=w2564:refnum<visa-resource-name>)  [unwired: 1 in, 2 out]
            n1757 = Concatenate Strings("cvolume" ("string"), "\r") -> (w2563:string)
            n1758 = VISA Write(VISA resource name=w2564, write buffer=w2563) -> (VISA resource name out=w2574:refnum<visa-resource-name>)  [unwired: 1 in, 2 out]
            n1759 = Concatenate Strings("irun" ("string"), "\r") -> (w2572:string)
            n1760 = VISA Write(VISA resource name=w2574, write buffer=w2572) -> ()  [unwired: 1 in, 3 out]
          }
          frame #1 {
            "Flushing P3" <- TRUE ("Flushing P3")
          }
        }
      }
      event "Flush Pump 1": Value Change {
        n1761 = event-data() -> ()  [unwired: 7 out]
        n1762 = flat-sequence {
          tunnel: [w2594] -> w2584
          tunnel: w2583 -> [w2587]
          tunnel: w2584 -> [_]
          frame #0 {
            # "set paramaters (rate, volume) for flush, clear volume"
            n1763 = local write "Inject Pump 1"(TRUE ("Inject Pump 1")) -> ()
            n1764 = Number To Decimal String(number="Flush rate (uL/m) P1") -> (decimal integer string=w2610:string)  [unwired: 1 in]
            n1765 = Concatenate Strings("irate  " ("string"), w2610, " u/m" ("string"), "\r") -> (w2612:string)
            n1766 = VISA Write(VISA resource name=w2587, write buffer=w2612) -> (VISA resource name out=w2608:refnum<visa-resource-name>)  [unwired: 1 in, 2 out]
            n1767 = Reciprocal(x="Flush rate (uL/m) P1") -> (1/x=w2591:dbl)
            n1768 = Number To Decimal String(number="Volume (uL) P1") -> (decimal integer string=w2599:string)  [unwired: 1 in]
            n1769 = Multiply(x="Volume (uL) P1", y=w2591) -> (x*y=w2590:dbl)
            n1770 = Concatenate Strings("tvolume  " ("string"), w2599, " u" ("string"), "\r") -> (w2597:string)
            n1771 = Multiply(x=w2590, y=60.0) -> (x*y=→"HP1 Flush Time (s)":dbl)
            n1772 = VISA Write(VISA resource name=w2608, write buffer=w2597) -> (VISA resource name out=w2596:refnum<visa-resource-name>)  [unwired: 1 in, 2 out]
            n1773 = Concatenate Strings("cvolume" ("string"), "\r") -> (w2595:string)
            n1774 = VISA Write(VISA resource name=w2596, write buffer=w2595) -> (VISA resource name out=w2606:refnum<visa-resource-name>)  [unwired: 1 in, 2 out]
            n1775 = Concatenate Strings("irun" ("string"), "\r") -> (w2604:string)
            n1776 = VISA Write(VISA resource name=w2606, write buffer=w2604) -> (VISA resource name out=w2594:refnum<visa-resource-name>)  [unwired: 1 in, 2 out]
          }
          frame #1 {
            "Flushing P1" <- TRUE ("Flushing P3")
          }
        }
      }
      event "Clear Volume": Value Change {
        n1777 = event-data() -> ()  [unwired: 7 out]
        n1778 = Concatenate Strings("cvolume" ("string"), "\r") -> (w2616:string)
        n1779 = VISA Write(VISA resource name=w2615, write buffer=w2616) -> ()  [unwired: 1 in, 3 out]
      }
      event "Clear Volume P3": Value Change {
        n1780 = event-data() -> ()  [unwired: 7 out]
        n1781 = Concatenate Strings("cvolume" ("string"), "\r") -> (w2622:string)
        n1782 = VISA Write(VISA resource name=w2621, write buffer=w2622) -> ()  [unwired: 1 in, 3 out]
        n1783 = local write "Clear Volume P3"(FALSE ("Clear Volume P3")) -> ()
      }
      event "Clear Volume P1": Value Change {
        n1784 = event-data() -> ()  [unwired: 7 out]
        n1785 = Concatenate Strings("cvolume" ("string"), "\r") -> (w2627:string)
        n1786 = local write "Clear Volume P1"(FALSE ("Clear Volume P1")) -> ()
        n1787 = VISA Write(VISA resource name=w2626, write buffer=w2627) -> ()  [unwired: 1 in, 3 out]
      }
      event "Display On P3": Value Change {
        n1788 = event-data() -> ()  [unwired: 7 out]
        n1789 = Select(t="dim 100", s="Display On P3", f="dim 0") -> (s? t:f=w2633:string)
        n1790 = Concatenate Strings(w2633, "\r") -> (w2635:string)
        n1791 = VISA Write(VISA resource name=w2630, write buffer=w2635) -> ()  [unwired: 1 in, 3 out]
      }
      event "Display On P1": Value Change {
        n1792 = event-data() -> ()  [unwired: 7 out]
        n1793 = Select(t="dim 100", s="Display On P1", f="dim 0") -> (s? t:f=w2640:string)
        n1794 = Concatenate Strings(w2640, "\r") -> (w2642:string)
        n1795 = VISA Write(VISA resource name=w2637, write buffer=w2642) -> ()  [unwired: 1 in, 3 out]
      }
      event "Retract Pump 3": Value Change {
        n1796 = event-data() -> ()  [unwired: 7 out]
        n1797 = local write "Retract Pump 3"(FALSE ("Retract Pump 3")) -> ()
        n1798 = case shown="True" "Retract Pump 3" {
          tunnel: w2644 -> [_ w2647]
          frame False {
          }
          frame True {
            n1799 = Number To Decimal String(number="Retract Rate (uL/m)") -> (decimal integer string=w2665:string)  [unwired: 1 in]
            n1800 = Concatenate Strings("wrate  " ("string"), w2665, " u/m" ("string"), "\r") -> (w2667:string)
            n1801 = VISA Write(VISA resource name=w2647, write buffer=w2667) -> (VISA resource name out=w2658:refnum<visa-resource-name>)  [unwired: 1 in, 2 out]
            n1802 = Number To Decimal String(number="Retract Vol 3 (uL)") -> (decimal integer string=w2660:string)  [unwired: 1 in]
            n1803 = Concatenate Strings("tvolume  " ("string"), w2660, " u" ("string"), "\r") -> (w2657:string)
            n1804 = VISA Write(VISA resource name=w2658, write buffer=w2657) -> (VISA resource name out=w2653:refnum<visa-resource-name>)  [unwired: 1 in, 2 out]
            n1805 = Concatenate Strings("cvolume" ("string"), "\r") -> (w2654:string)
            n1806 = VISA Write(VISA resource name=w2653, write buffer=w2654) -> (VISA resource name out=w2648:refnum<visa-resource-name>)  [unwired: 1 in, 2 out]
            n1807 = Concatenate Strings("wrun" ("string"), "\r") -> (w2649:string)
            n1808 = VISA Write(VISA resource name=w2648, write buffer=w2649) -> ()  [unwired: 1 in, 3 out]
          }
        }
      }
      event "Retract Pump 1": Value Change {
        n1809 = event-data() -> ()  [unwired: 7 out]
        n1810 = local write "Retract Pump 1"(FALSE ("Retract Pump 1")) -> ()
        n1811 = case shown="True" "Retract Pump 1" {
          tunnel: w2669 -> [_ w2674]
          frame False {
          }
          frame True {
            n1812 = local read "Retract Rate (uL/m)"() -> (w2672:dbl)
            n1813 = Number To Decimal String(number=w2672) -> (decimal integer string=w2690:string)  [unwired: 1 in]
            n1814 = Concatenate Strings("wrate  " ("string"), w2690, " u/m" ("string"), "\r") -> (w2692:string)
            n1815 = VISA Write(VISA resource name=w2674, write buffer=w2692) -> (VISA resource name out=w2684:refnum<visa-resource-name>)  [unwired: 1 in, 2 out]
            n1816 = Number To Decimal String(number="Retract Vol 1 (uL)") -> (decimal integer string=w2686:string)  [unwired: 1 in]
            n1817 = Concatenate Strings("tvolume  " ("string"), w2686, " u" ("string"), "\r") -> (w2683:string)
            n1818 = VISA Write(VISA resource name=w2684, write buffer=w2683) -> (VISA resource name out=w2680:refnum<visa-resource-name>)  [unwired: 1 in, 2 out]
            n1819 = Concatenate Strings("cvolume" ("string"), "\r") -> (w2681:string)
            n1820 = VISA Write(VISA resource name=w2680, write buffer=w2681) -> (VISA resource name out=w2675:refnum<visa-resource-name>)  [unwired: 1 in, 2 out]
            n1821 = Concatenate Strings("wrun" ("string"), "\r") -> (w2676:string)
            n1822 = VISA Write(VISA resource name=w2675, write buffer=w2676) -> ()  [unwired: 1 in, 3 out]
          }
        }
      }
      event "Flip Green Filter": Value Change {
        n1823 = event-data() -> ()  [unwired: 7 out]
        n1824 = Not(x="Flip Green Filter") -> (.not. x?=w2694:bool)
        n1825 = local write "Flip Green Filter"(w2694) -> ()
        n1826 = flat-sequence {
          tunnel: w2702 -> [w2707]
          tunnel: w2701 -> [w2706]
          tunnel: [w2704] -> w2699
          tunnel: [w2703] -> w2698
          tunnel: [w2709] -> w2697
          tunnel: w2699 -> [w2709]
          tunnel: [w2708] -> w2696
          tunnel: w2698 -> [w2708]
          tunnel: w2697 -> [w2713]
          tunnel: w2696 -> [w2712]
          tunnel: [w2711] -> w2700
          frame #0 {
            n1827 = xnode "Read/Write Control"("FPGA VI Reference In"=w2707, "error in"=w2706, "Green Filter Flipper"=TRUE) -> ("FPGA VI Reference Out"=w2704:T20, "error out"=w2703:errorcluster)
          }
          frame #1 {
            n1828 = Wait (ms)(milliseconds to wait=u32 100) -> ()  [unwired: 1 out]
          }
          frame #2 {
            n1829 = xnode "Read/Write Control"("FPGA VI Reference In"=w2713, "error in"=w2712, "Green Filter Flipper"=FALSE) -> ("error out"=w2711:errorcluster)  [unwired: 1 out]
          }
        }
      }
      event "Pump 1 contents", "Pump 3 contents": Value Change {
        n1830 = event-data() -> ()  [unwired: 7 out]
        n1831 = local read "Pump 1 contents"() -> (→"Pump 1 cont disp":string)
        n1832 = local read "Pump 3 contents"() -> (→"Pump 3 cont disp":string)
      }
      event "Reset Trap Pos. FB": Value Change {
        n1833 = event-data() -> ()  [unwired: 7 out]
        n1834 = xnode "Read/Write Control"("FPGA VI Reference In"=w2719, "error in"=w2718, "Trap Pos. FB Reset"="Reset Trap Pos. FB") -> ()  [unwired: 2 out]
      }
      event "Rem fb disp offset": Value Change {
        n1835 = event-data() -> ()  [unwired: 7 out]
        n1836 = local write "Rem fb disp offset"(FALSE ("Rem fb disp offset")) -> ()
        n1837 = local read "Mean T1 Position (nm)"() -> (w2721:dbl)
        n1838 = local read "FB Trap Pos Offset"() -> (w2722:dbl)
        n1839 = Subtract(x=w2722, y=w2721) -> (x-y=w2720:dbl)
        n1840 = local write "FB Trap Pos Offset"(w2720) -> ()
      }
      event "Threshold (nm)": Value Change {
        n1841 = event-data() -> ()  [unwired: 7 out]
        n1842 = flat-sequence {
          tunnel: w2726 -> [w2734]
          tunnel: w2725 -> [w2733]
          tunnel: [w2727] -> w2724
          tunnel: w2724 -> [w2740]
          frame #0 {
            n1843 = xnode "Read/Write Control"("FPGA VI Reference In"=w2734, "error in"=w2733) -> ("FPGA VI Reference Out"=w2730:T20, "error out"=w2729:errorcluster, "FPGA TTrig Thresh"=w2731:i64)
            n1844 = local read "Threshold stored (nm)"() -> (w2739:dbl)
            n1845 = local read "Threshold (nm)"() -> (w2727:dbl)
            n1846 = local read "AOM X Cal (nm/MHz)"() -> (w2737:dbl)
            n1847 = Subtract(x=w2727, y=w2739) -> (x-y=w2738:dbl)
            n1848 = Divide(x=w2738, y=w2737) -> (x/y=w2735:dbl)
            n1849 = call "IR AOM freq to word.vi"("Frequency In (MHz)"=w2735) -> ("Frequency Word Out (double)"=w2736:dbl)
            n1850 = To Quad Integer(1:w2736) -> (0:w2732:i64)
            n1851 = Add(x=w2731, y=w2732) -> (x+y=w2728:i64)
            n1852 = xnode "Read/Write Control"("FPGA VI Reference In"=w2730, "error in"=w2729, "FPGA TTrig Thresh"=w2728) -> ()  [unwired: 2 out]
          }
          frame #1 {
